vi "仪器参数设置.vi"(11 "仪器参数设置输入":T1(array[cluster]) {"单位" items=["ug/L", "mg/L"]}) -> (2 "确定":bool, 3 "仪器参数设置输出":T1(array[cluster]) {"单位" items=["ug/L", "mg/L"]})   [LabVIEW 2016, in "斯坦道多参数.lvlib"]
uses:
  <vilib>/Utility/miscctls.llb/LVPointTypeDef.ctl
panel:
  in  "多参数":enum16{"pH", "水温", "电导率", "溶解氧", "浊度"}(ring)
  in  "单位":enum16{"ug/L", "mg/L"}(ring)
  in  "标样校准时间":timestamp
  in  "二次多项式系数":dbl
  in  "线性相关系数":dbl
  in  "测量信号值":dbl
  in  "测量检出限":dbl
  in  "曲线斜率":dbl
  in  "曲线截距":dbl
  in  "空白校准时间":timestamp
  in  "消解时长":dbl
  in  "消解温度":dbl
  in  "测量间隔":dbl
  in  "测量精度":dbl
  in  "测量量程":dbl
  in  "取消":bool
  in  "确定":bool
  # "仪器参数设置"
  # "多参数"
  # "监测参数"
  # "黑色框参数需要手动输入\n灰色框参数自动读取不需要手动输入"
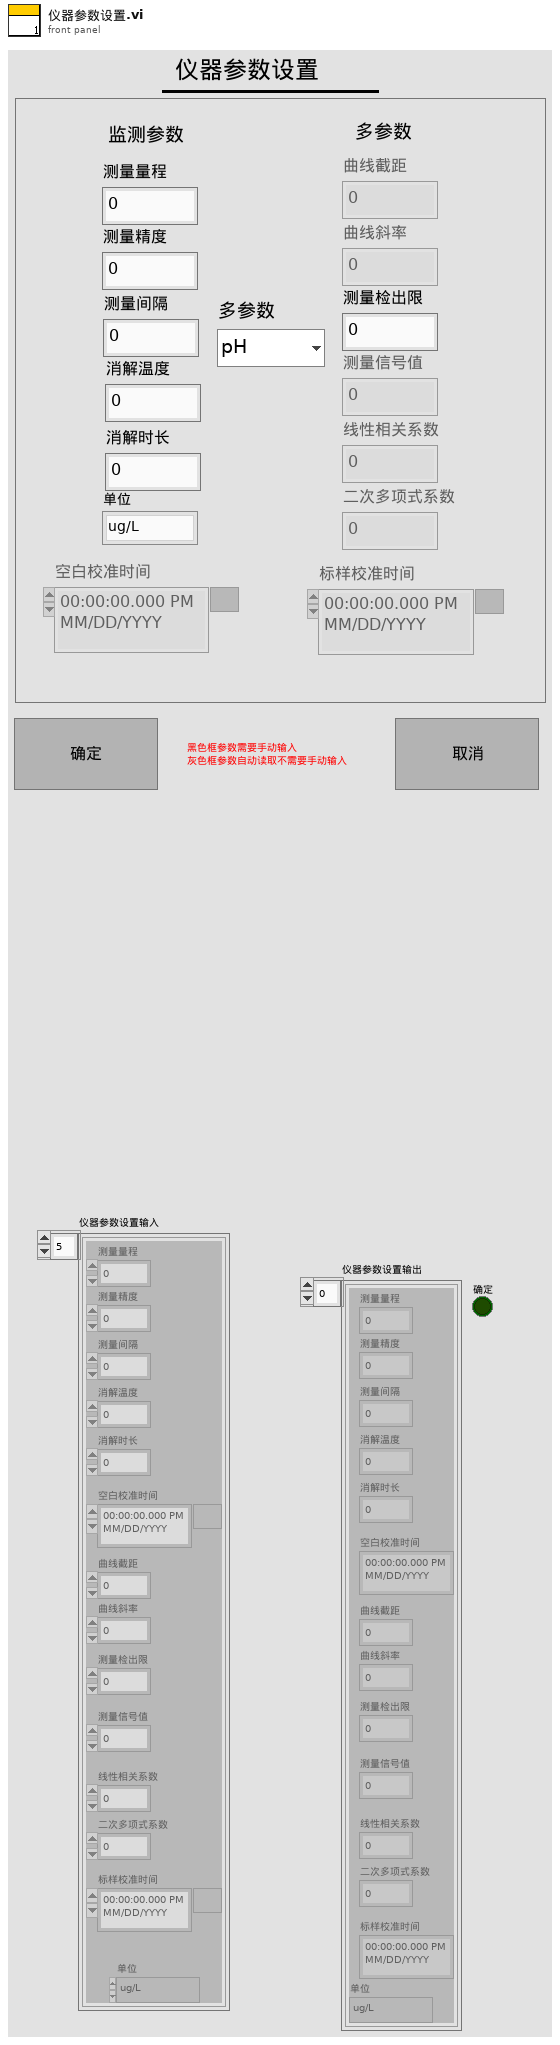
[diagram p1: front panel]
types:
  T1 = cluster{"测量量程":dbl, "测量精度":dbl, "测量间隔":dbl, "消解温度":dbl, "消解时长":dbl, "空白校准时间":timestamp, "曲线截距":dbl, "曲线斜率":dbl, "测量检出限":dbl, "测量信号值":dbl, "线性相关系数":dbl, "二次多项式系数":dbl, "标样校准时间":timestamp, "单位":u16}[]
  T2 = typedef "LVPointTypeDef.ctl" = cluster{"Horizontal":i16, "Vertical":i16}
  T3 = cluster{"测量量程":dbl, "测量精度":dbl, "测量间隔":dbl, "消解温度":dbl, "消解时长":dbl, "空白校准时间":timestamp, "曲线截距":dbl, "曲线斜率":dbl, "测量检出限":dbl, "测量信号值":dbl, "线性相关系数":dbl, "二次多项式系数":dbl, "标样校准时间":timestamp, "单位":u16}
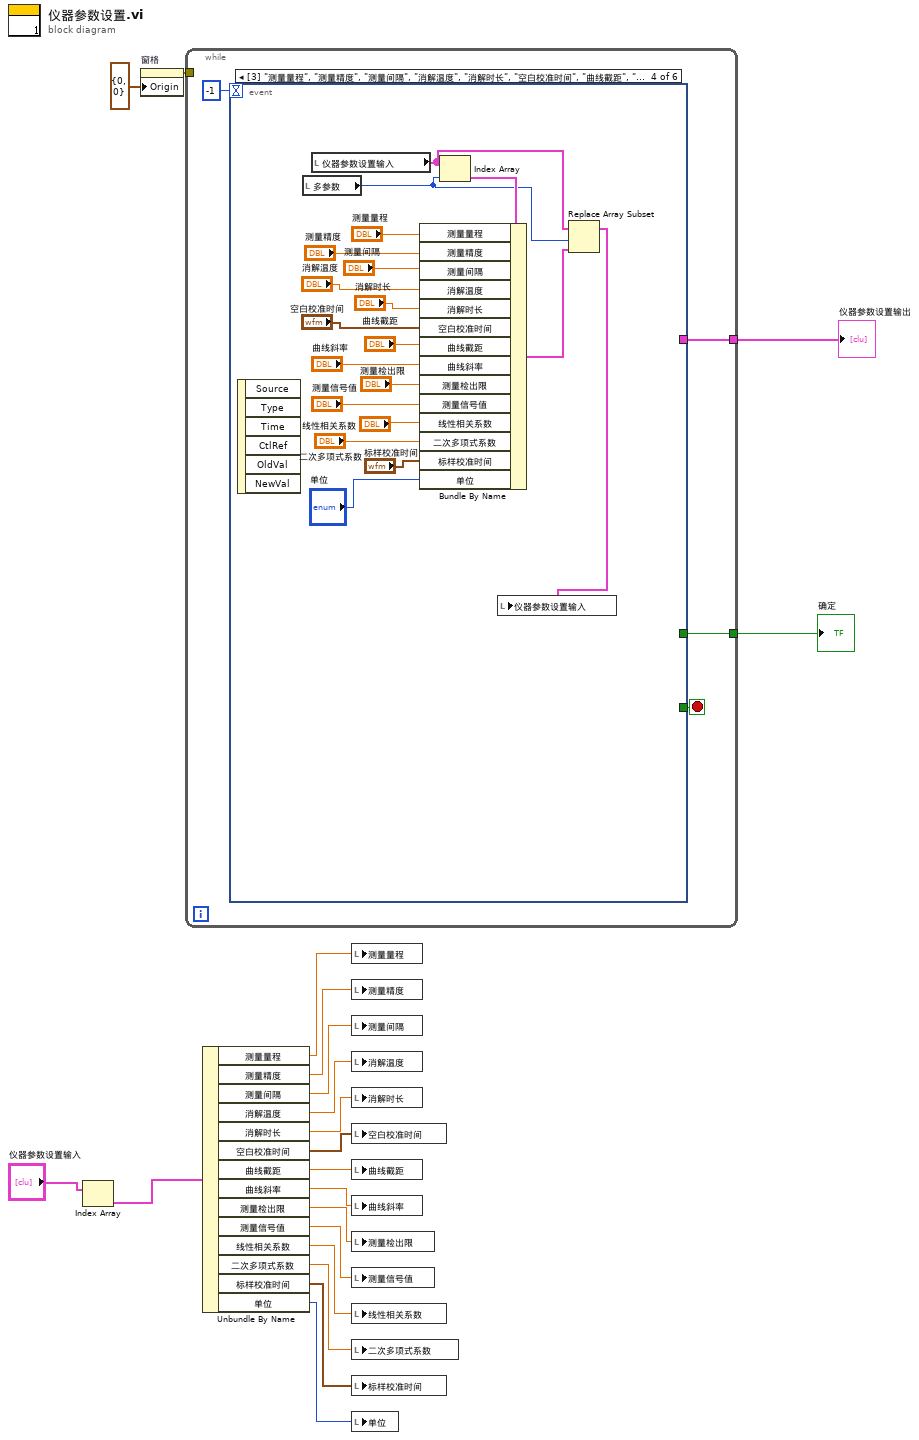
[diagram p0: block diagram]
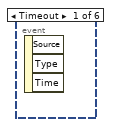
[diagram p2: hidden frame]
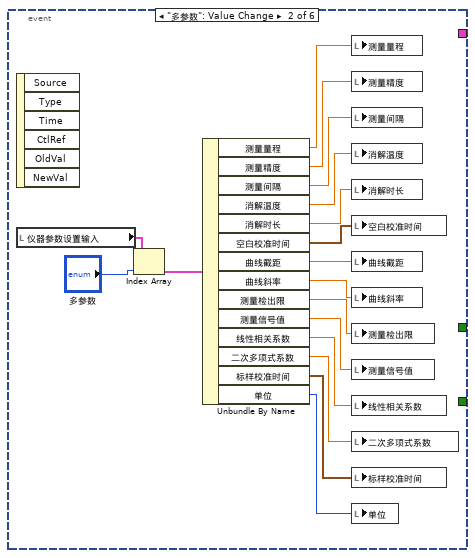
[diagram p3: hidden frame]
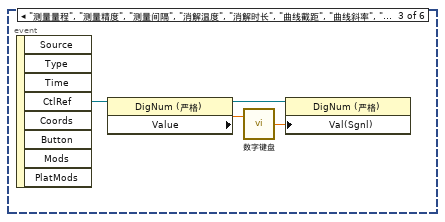
[diagram p4: hidden frame]
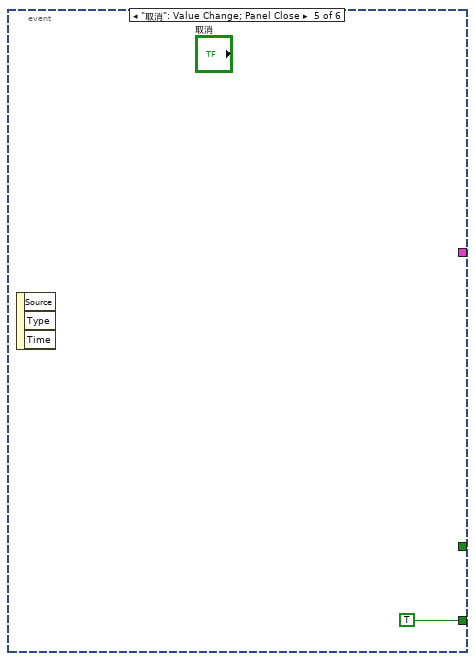
[diagram p5: hidden frame]
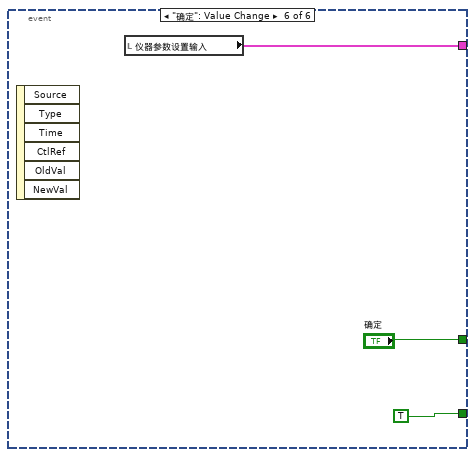
[diagram p6: hidden frame]
diagram:
  n1 = Index Array(array="仪器参数设置输入") -> (element=w3:T3)  [unwired: 1 in]
  n2 = property on="窗格" class="Pane"("Origin"=T2 {"Horizontal"=0, "Vertical"=0} ("原点")) -> (error out=w19:errorcluster)  [unwired: 2 in, 1 out]
  n3 = while {
    tunnel: w19 -> [_]
    tunnel: [w23] -> w2
    tunnel: [w22] -> w1
    stop <- w24 stop-if-true
    n4 = event shown="[3] \"测量量程\", \"测量精度\", \"测量间隔\", \"消解温度\", \"消解时长\", \"空白校准时间\", \"曲线截距\", \"曲线斜率\", \"测量检出限\", \"测量信号值\", \"线性相关系数\", \"二次多项式系数\", \"标样校准时间\": 值改变" {
      selector: _ -> [_ _ _ _ _ _]
      dyn-events: _ -> [_ _ _ _ _ _]
      timeout: -1 -> [_ _ _ _ _ _]
      tunnel: [_ _ _ _ TRUE TRUE] -> w24
      tunnel: [_ _ _ _ _ "确定"] -> w23
      tunnel: [_ _ _ _ _ w66] -> w22
      event Timeout {
        n5 = event-data() -> ()  [unwired: 1 in, 3 out]
      }
      event "多参数": Value Change {
        n6 = event-data() -> ()  [unwired: 1 in, 6 out]
        n7 = local read "仪器参数设置输入"() -> (w26:T1)
        n8 = Index Array(array=w26, index="多参数") -> (element=w41:T3)
        n9 = Unbundle By Name(w41) -> ("测量量程"=w27:dbl, "测量精度"=w28:dbl, "测量间隔"=w29:dbl, "消解温度"=w30:dbl, "消解时长"=w31:dbl, "空白校准时间"=w32:timestamp, "曲线截距"=w33:dbl, "曲线斜率"=w34:dbl, "测量检出限"=w35:dbl, "测量信号值"=w36:dbl, "线性相关系数"=w37:dbl, "二次多项式系数"=w38:dbl, "标样校准时间"=w39:timestamp, "单位"=w40:u16)
        n10 = local write "测量量程"(w27) -> ()
        n11 = local write "测量精度"(w28) -> ()
        n12 = local write "测量间隔"(w29) -> ()
        n13 = local write "消解温度"(w30) -> ()
        n14 = local write "消解时长"(w31) -> ()
        n15 = local write "空白校准时间"(w32) -> ()
        n16 = local write "曲线截距"(w33) -> ()
        n17 = local write "曲线斜率"(w34) -> ()
        n18 = local write "测量检出限"(w35) -> ()
        n19 = local write "测量信号值"(w36) -> ()
        n20 = local write "线性相关系数"(w37) -> ()
        n21 = local write "二次多项式系数"(w38) -> ()
        n22 = local write "标样校准时间"(w39) -> ()
        n23 = local write "单位"(w40) -> ()
      }
      event "测量量程", "测量精度", "测量间隔", "消解温度", "消解时长", "曲线截距", "曲线斜率", "测量检出限", "测量信号值", "线性相关系数", "二次多项式系数": Mouse Down {
        n24 = event-data() -> ("CtlRef"=w42:refnum<vi>)  [unwired: 1 in, 7 out]
        n25 = property class="DigNum (严格)"(reference=w42) -> (reference out=w44:refnum<vi>, "Value"=w45:dbl)  [unwired: 1 in, 1 out]
        n26 = call "数字键盘.vi"("OldNumber"=w45) -> ("NewNumber"=w43:dbl)  [unwired: 1 in]
        n27 = property class="DigNum (严格)"(reference=w44, "Val(Sgnl)"=w43) -> ()  [unwired: 1 in, 2 out]
      }
      event "测量量程", "测量精度", "测量间隔", "消解温度", "消解时长", "空白校准时间", "曲线截距", "曲线斜率", "测量检出限", "测量信号值", "线性相关系数", "二次多项式系数", "标样校准时间": Value Change {
        n28 = event-data() -> ()  [unwired: 1 in, 6 out]
        n29 = local read "多参数"() -> (w62:enum16{"pH", "水温", "电导率", "溶解氧", "浊度"})
        n30 = local read "仪器参数设置输入"() -> (w63:T1)
        n31 = Index Array(array=w63, index=w62) -> (element=w64:T3)
        n32 = Bundle By Name(cluster=w64, "测量量程"="测量量程", "测量精度"="测量精度", "测量间隔"="测量间隔", "消解温度"="消解温度", "消解时长"="消解时长", "空白校准时间"="空白校准时间", "曲线截距"="曲线截距", "曲线斜率"="曲线斜率", "测量检出限"="测量检出限", "测量信号值"="测量信号值", "线性相关系数"="线性相关系数", "二次多项式系数"="二次多项式系数", "标样校准时间"="标样校准时间", "单位"="单位") -> (w61:T3)
        n33 = Replace Array Subset(array=w63, new element=w61, index=w62) -> (w60:T1)
        n34 = local write "仪器参数设置输入"(w60) -> ()
      }
      event "取消": Value Change; Panel Close {
        n35 = event-data() -> ()  [unwired: 1 in, 3 out]
      }
      event "确定": Value Change {
        n36 = event-data() -> ()  [unwired: 1 in, 6 out]
        n37 = local read "仪器参数设置输入"() -> (w66:T1)
      }
    }
  }
  "仪器参数设置输出" <- w1
  "确定" <- w2
  n38 = Unbundle By Name(w3) -> ("测量量程"=w18:dbl, "测量精度"=w17:dbl, "测量间隔"=w16:dbl, "消解温度"=w15:dbl, "消解时长"=w14:dbl, "空白校准时间"=w13:timestamp, "曲线截距"=w12:dbl, "曲线斜率"=w11:dbl, "测量检出限"=w10:dbl, "测量信号值"=w9:dbl, "线性相关系数"=w8:dbl, "二次多项式系数"=w7:dbl, "标样校准时间"=w6:timestamp, "单位"=w5:u16)
  n39 = local write "测量量程"(w18) -> ()
  n40 = local write "测量精度"(w17) -> ()
  n41 = local write "测量间隔"(w16) -> ()
  n42 = local write "消解温度"(w15) -> ()
  n43 = local write "消解时长"(w14) -> ()
  n44 = local write "空白校准时间"(w13) -> ()
  n45 = local write "曲线截距"(w12) -> ()
  n46 = local write "曲线斜率"(w11) -> ()
  n47 = local write "测量检出限"(w10) -> ()
  n48 = local write "测量信号值"(w9) -> ()
  n49 = local write "线性相关系数"(w8) -> ()
  n50 = local write "二次多项式系数"(w7) -> ()
  n51 = local write "标样校准时间"(w6) -> ()
  n52 = local write "单位"(w5) -> ()
